vi "Close.vi"(8 "error in (no error)":errorcluster {"code" format="Error %.0f"}, 11 "Progress Bar UI In":refnum<class "Progress Bar UI.lvclass">) -> (0 "error out":errorcluster {"code" format="Error %.0f"})   [LabVIEW 2023, in "Progress Bar UI.lvclass"]
uses:
  Progress Bar UI.lvclass
  Progress Bar UI.lvclass/Progress Bar UI.ctl
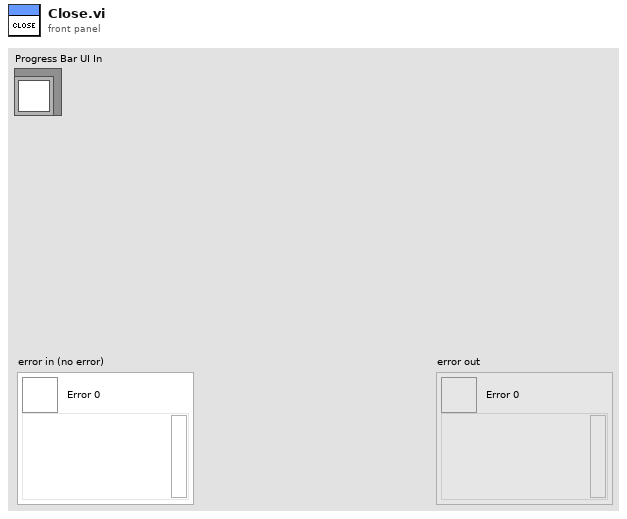
[diagram p1: front panel]
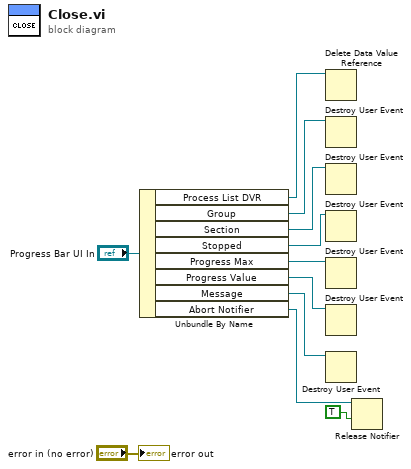
[diagram p0: block diagram]
diagram:
  n1 = Unbundle By Name("Progress Bar UI In") -> ("Process List DVR"=w2:refnum<data-value>, "Group"=w3:refnum<user-event>, "Section"=w4:refnum<user-event>, "Stopped"=w5:refnum<user-event>, "Progress Max"=w6:refnum<user-event>, "Progress Value"=w7:refnum<user-event>, "Message"=w8:refnum<user-event>, "Abort Notifier"=w10:refnum<notifier>)
  n2 = Delete Data Value Reference(data value reference=w2) -> ()  [unwired: 1 in, 2 out]
  n3 = Destroy User Event(user event=w3) -> ()  [unwired: 1 in, 1 out]
  n4 = Destroy User Event(user event=w4) -> ()  [unwired: 1 in, 1 out]
  n5 = Destroy User Event(user event=w5) -> ()  [unwired: 1 in, 1 out]
  n6 = Destroy User Event(user event=w6) -> ()  [unwired: 1 in, 1 out]
  n7 = Destroy User Event(user event=w7) -> ()  [unwired: 1 in, 1 out]
  n8 = Destroy User Event(user event=w8) -> ()  [unwired: 1 in, 1 out]
  n9 = Release Notifier(notifier=w10, force destroy? (F)=TRUE) -> ()  [unwired: 1 in, 3 out]
  "error out" <- "error in (no error)"
